vi "GetPositionCategory.vi"(8 "error in (no error)":errorcluster, 11 "Link in":refnum<class "Link.lvclass">) -> (0 "error out":errorcluster, 2 "position":T1, 3 "Link out":refnum<class "Link.lvclass">)   [LabVIEW 2009, in "NavScreen.lvlib" / "Link.lvclass"]
uses:
  Link.lvclass
  PositionCategory.ctl
  NavScreen.lvlib
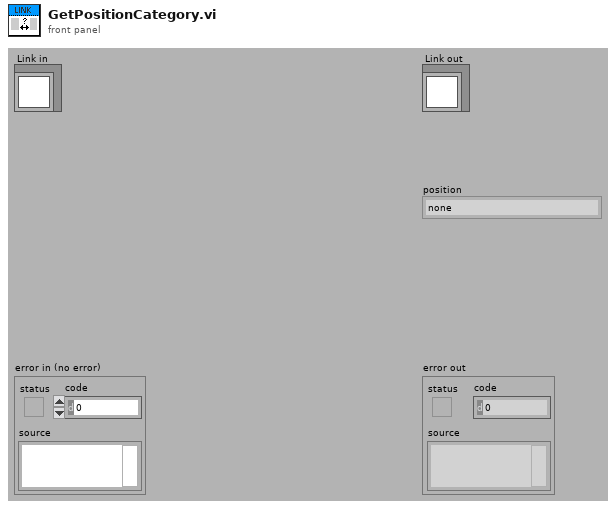
[diagram p1: front panel]
types:
  T1 = typedef "NavScreen.lvlib/PositionCategory.ctl" = enum16{"none", "column 1", "column 2", "ring"}
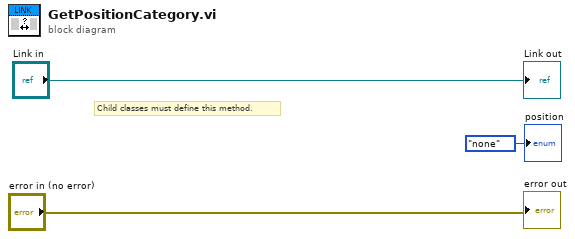
[diagram p0: block diagram]
diagram:
  # "Child classes must define this method."
  "error out" <- "error in (no error)"
  "Link out" <- "Link in"
  "position" <- PositionCategory."none" ("position")
